vi "ParseArgumentsCore.vi"(8 "error in (no error)":errorcluster, 9 "Value":string, 10 "Option":string, 11 "ExecuteBuildSpecAllTargets in":refnum<class "ExecuteBuildSpecAllTargets.lvclass">) -> (0 "error out":errorcluster, 3 "ExecuteBuildSpecAllTargets out":refnum<class "ExecuteBuildSpecAllTargets.lvclass">)   [LabVIEW 2023, in "ExecuteBuildSpecAllTargets.lvclass"]
doc: "Parses command line arguments passed through LabVIEWCLI."
uses:
  ExecuteBuildSpecAllTargets.lvclass
  ExecuteBuildSpecAllTargets.lvclass/ExecuteBuildSpecAllTargets.ctl
  C:/Program Files (x86)/National Instruments/Shared/LabVIEW CLI/Operations/Utilities/OperationErrorType.ctl
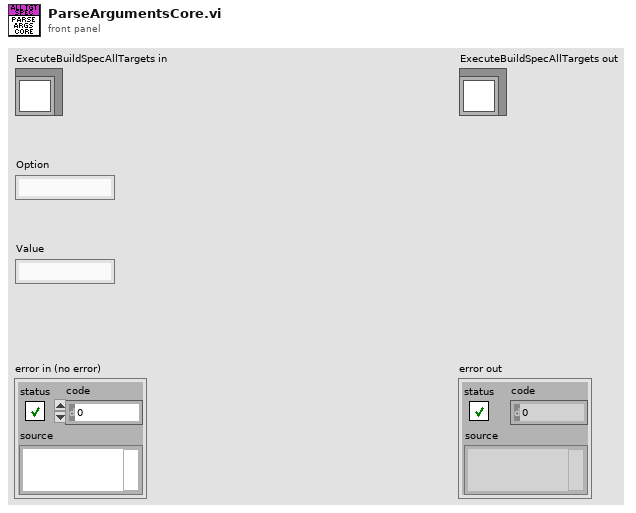
[diagram p1: front panel]
types:
  T1 = typedef "OperationErrorType.ctl" = enum16{"RequiredArgumentMissing", "UnknownArguments", "LoggerSetMultipleTimes", "OperationBrokenError"}
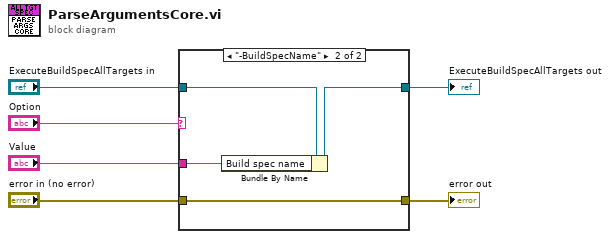
[diagram p0: block diagram]
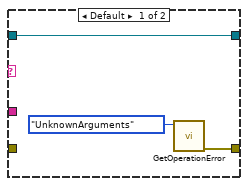
[diagram p2: hidden frame]
diagram:
  n1 = case shown="\"-BuildSpecName\"" "Option" {
    tunnel: "error in (no error)" -> [_ w13]
    tunnel: [w7 w13] -> w2
    tunnel: "Value" -> [_ w12]
    tunnel: "ExecuteBuildSpecAllTargets in" -> [w9 w11]
    tunnel: [w9 w10] -> w3
    frame Default {
      n2 = call "GetOperationError.vi"("Operation Error Type"=OperationErrorType."UnknownArguments") -> ("error out"=w7:errorcluster)  [unwired: 10 in]
    }
    frame "-BuildSpecName" {
      n3 = Bundle By Name(cluster=w11, "Build spec name"=w12) -> (w10:refnum<class "ExecuteBuildSpecAllTargets.lvclass">)
    }
  }
  "error out" <- w2
  "ExecuteBuildSpecAllTargets out" <- w3
